vi "TSM DAQmx Relay Write.vi"(8 "error in":errorcluster, 9 "Pins to Output LOW":tag[](array[tag]), 10 "Pins to Output HIGH":tag[](array[tag]), 11 "TSM context in":T1) -> (0 "error out":errorcluster, 3 "TSM context out":T1)   [LabVIEW 2019]
uses:
  <vilib>/NI_TestStand_SemiconductorModule/NI_TestStand_Semiconductor_Module.lvlibp/PinMap/General/SemiconductorModuleContext.ctl
  <vilib>/NI_TestStand_SemiconductorModule/NI_TestStand_Semiconductor_Module.lvlibp/PinMap/General/NIInstrumentTypeIDs.ctl
  <vilib>/DAQmx/write.llb/DAQmx Write (Digital 1D Bool 1Chan 1Samp).vi
  <vilib>/NI_TestStand_SemiconductorModule/NI_TestStand_Semiconductor_Module.lvlibp/PinMap/DAQmx/PinsToNIDAQmxTasks.vi
  <vilib>/DAQmx/miscellaneous.llb/DAQmx Fill In Error Info.vi
  <vilib>/NI_TestStand_SemiconductorModule/NI_TestStand_Semiconductor_Module.lvlibp
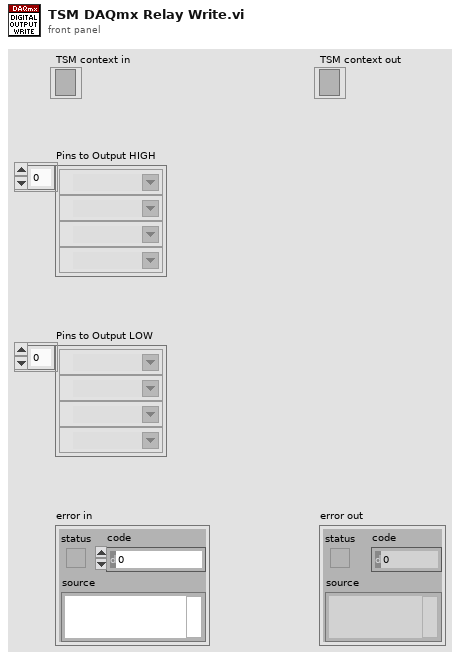
[diagram p1: front panel]
types:
  T1 = typedef "NI_TestStand_Semiconductor_Module.lvlibp/SemiconductorModuleContext.ctl" = refnum<k7>
  T2 = typedef "NI_TestStand_Semiconductor_Module.lvlibp/NIInstrumentTypeIDs.ctl" = string
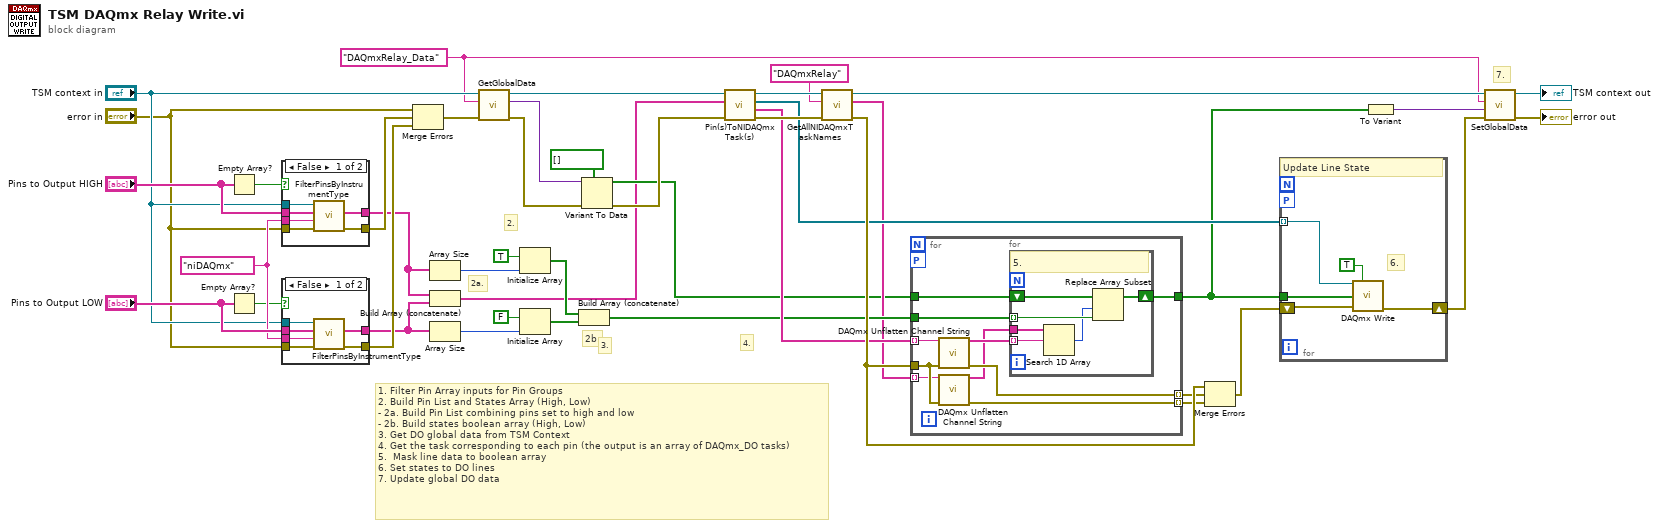
[diagram p0: block diagram]
diagram:
  w14 = T2 "niDAQmx" ("Instrument Type Id")
  w4 = "DAQmxRelay_Data" ("Data Id")
  # "7."
  # "2b."
  # "2a."
  # "1. Filter Pin Array inputs for Pin Groups\n2. Build Pin List and States Array (High, Low)\n- 2a. Build Pin List combining pins set to high and low\n- 2b. Build states boolean array (High, Low)\n3. Get DO global data from TSM Context\n4. Get the task corresponding to each pin (the output is an array of DAQmx_DO tasks)\n5.  Mask line data to boolean array\n6. Set states to DO lines\n7. Update global DO data"
  # "4."
  # "3."
  # "2."
  n1 = Empty Array?(array="Pins to Output HIGH") -> (empty?=w32:bool)
  n2 = Empty Array?(array="Pins to Output LOW") -> (empty?=w13:bool)
  n3 = case shown="False" w32 {
    tunnel: "Pins to Output HIGH" -> [w49 w50]
    tunnel: [w48 w50] -> w18
    tunnel: [w47 w51] -> w30
    tunnel: "error in" -> [w46 w51]
    tunnel: "TSM context in" -> [w45 _]
    tunnel: w14 -> [w44 _]
    frame False {
      n4 = call <vilib>:"FilterPinsByInstrumentType.vi"("error in (no error)"=w46, "Instrument Type Id"=w44, "Pins"=w49, "Semiconductor Module Context"=w45) -> ("error out"=w47:errorcluster, "Filtered Pins"=w48:tag[])  [unwired: 5 in, 1 out]
    }
    frame True {
    }
  }
  n5 = case shown="False" w13 {
    tunnel: "Pins to Output LOW" -> [w57 w58]
    tunnel: [w56 w58] -> w17
    tunnel: [w55 w59] -> w33
    tunnel: "error in" -> [w54 w59]
    tunnel: "TSM context in" -> [w53 _]
    tunnel: w14 -> [w52 _]
    frame False {
      n6 = call <vilib>:"FilterPinsByInstrumentType.vi"("error in (no error)"=w54, "Instrument Type Id"=w52, "Pins"=w57, "Semiconductor Module Context"=w53) -> ("error out"=w55:errorcluster, "Filtered Pins"=w56:tag[])  [unwired: 5 in, 1 out]
    }
    frame True {
    }
  }
  n7 = Merge Errors("error in", w30, w33) -> (w34:errorcluster)
  n8 = Array Size(array=w18) -> (size(s)=w22:i32)
  n9 = Build Array (concatenate)(w18, w17) -> (w3:tag[])
  n10 = Array Size(array=w17) -> (size(s)=w21:i32)
  n11 = call <vilib>:"GetGlobalData.vi"("error in (no error)"=w34, "Data Id"=w4, "Semiconductor Module Context"="TSM context in") -> ("error out"=w42:errorcluster, "Data"=w41:variant, "Semiconductor Module Context Out"=w6:T1)  [unwired: 6 in]
  n12 = Initialize Array(TRUE, w22) -> (w15:bool[])
  n13 = Initialize Array(FALSE ("element"), w21) -> (w19:bool[])
  n14 = Build Array (concatenate)(w15, w19) -> (w16:bool[])
  n15 = Variant To Data(error in=w42, type=bool[] [], Variant=w41) -> (data=w5:bool[], error out=w40:errorcluster)
  n16 = call-poly <vilib>:"Pin(s)ToNIDAQmxTask(s).vi"("error in (no error)"=w40, "Pins"=w3, "Semiconductor Module Context"=w6) -> ("error out"=w37:errorcluster, "Channel Lists"=w28:string[], "DAQmx Tasks"=w25:refnum<k21>[], "Semiconductor Module Context Out"=w38:T1)  [unwired: 4 in, 1 out]
  n17 = call <vilib>:"GetAllNIDAQmxTaskNames.vi"("error in (no error)"=w37, "Task Type"="DAQmxRelay", "Semiconductor Module Context"=w38) -> ("error out"=w43:errorcluster, "Channel Lists"=w11:string[], "Semiconductor Module Context Out"=w24:T1)  [unwired: 5 in, 1 out]
  n18 = for {
    tunnel: w5 -> [w67]
    tunnel: [w66] -> w2
    tunnel: w16 -> [w65]
    tunnel: w11 -> [w64] mode=indexing
    tunnel: w28 -> [w63] mode=indexing
    tunnel: w43 -> [w69]
    tunnel: [w61] -> w36 mode=indexing
    workers-P: _ -> [_]
    tunnel: [w62] -> w35 mode=indexing
    n19 = call <vilib>:"DAQmx Unflatten Channel String.vi"("names in"=w63, "error in"=w69) -> ("names out"=w68:string[], "error out"=w62:errorcluster)  [unwired: 12 in]
    n20 = call <vilib>:"DAQmx Unflatten Channel String.vi"("names in"=w64, "error in"=w69) -> ("names out"=w60:string[], "error out"=w61:errorcluster)  [unwired: 12 in]
    n21 = for {
      tunnel: w60 -> [w75]
      tunnel: w68 -> [w74] mode=indexing
      tunnel: w65 -> [w71] mode=indexing
      shift-right: [w72] -> w66
      shift-left: w67 -> [w73]
      # "5."
      n22 = Search 1D Array(1D array=w75, element=w74) -> (index of element=w70:i32)  [unwired: 1 in]
      n23 = Replace Array Subset(array=w73, new element=w71, index=w70) -> (w72:bool[])
    }
  }
  n24 = Merge Errors(w43, w35, w36) -> (w26:errorcluster)
  n25 = for {
    tunnel: w2 -> [w77]
    tunnel: w25 -> [w79] mode=indexing
    workers-P: _ -> [_]
    shift-right: [w76] -> w8
    shift-left: w26 -> [w80]
    # "6."
    # "Update Line State"
    n26 = call-poly <vilib>:"DAQmx Write.vi"("task/channels in"=w79, "auto start"=TRUE, "data"=w77, "error in"=w80) -> ("error out"=w76:errorcluster)  [unwired: 9 in, 2 out]
  }
  n27 = To Variant(anything=w2) -> (Variant=w1:variant)
  n28 = call <vilib>:"SetGlobalData.vi"("error in (no error)"=w8, "Data"=w1, "Data Id"=w4, "Semiconductor Module Context"=w24) -> ("error out"=→"error out":errorcluster, "Semiconductor Module Context Out"=→"TSM context out":T1)  [unwired: 5 in]
